vi "Target Color.vi"() -> (3 "Color":string)   [LabVIEW 2019]
uses:
  <vilib>/numeric/sub_Random U32.vi
  <vilib>/numeric/Random Number (Range) U64.vi
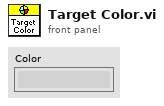
[diagram p1: front panel]
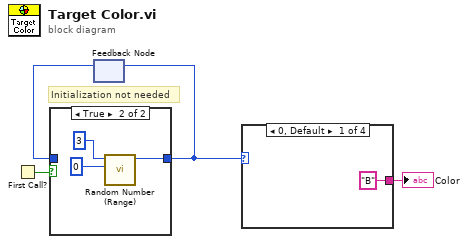
[diagram p0: block diagram]
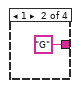
[diagram p3: hidden frame]
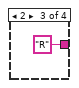
[diagram p4: hidden frame]
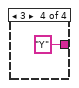
[diagram p5: hidden frame]
diagram:
  # "Initialization not needed"
  n1 = First Call?() -> (First Call?: T/F=w3:bool)
  n2 = feedback #1() -> (w1:u64)  [unwired: 1 in]
  n3 = case shown="True" w3 {
    tunnel: [w5 w6] -> w2
    tunnel: w1 -> [w5 _]
    frame False {
    }
    frame True {
      n4 = call-poly <vilib>:"Random Number (Range).vi"("lower bound (0)"=u64 0, "upper bound (100)"=u64 3) -> ("number"=w6:u64)  [unwired: 9 in]
    }
  }
  n5 = feedback-in #1(w2) -> ()
  n6 = case shown="0, Default" w2 {
    tunnel: ["B" "G" "R" "Y"] -> w4
    frame 0, Default {
    }
    frame 1 {
    }
    frame 2 {
    }
    frame 3 {
    }
  }
  "Color" <- w4
